vi "Write.vi"(8 "Error In":errorcluster, 9 "Data":u8[](array[numeric]), 10 "Command":u8, 11 "EZ430-Chronos Config":T1) -> (0 "Error Out":errorcluster, 3 "EZ430-Chronos Config":T1)   [LabVIEW 2011, in "LVH-EZ430.lvlib"]
uses:
  <vilib>/LabVIEW Hacker/LabVIEW Interface for EZ430-Chronos/LVH-EZ430.lvlib
  <vilib>/LabVIEW Hacker/LabVIEW Interface for EZ430-Chronos/Private/Type Defs/EZ430-Chronos Ref.ctl
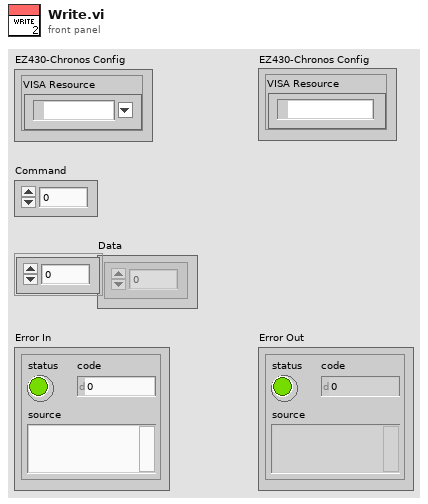
[diagram p1: front panel]
types:
  T1 = typedef "LVH-EZ430.lvlib/EZ430-Chronos Ref.ctl" = cluster{"VISA Resource":refnum<visa-resource-name>}
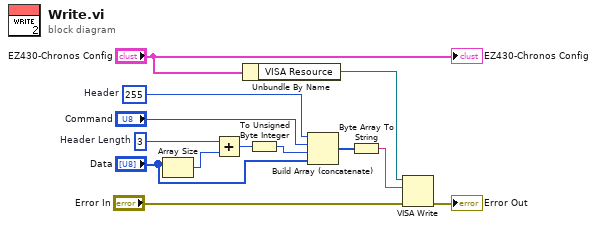
[diagram p0: block diagram]
diagram:
  w10 = 3  # Header Length
  w13 = u8 255  # Header
  n1 = Array Size(array="Data") -> (size(s)=w11:i32)
  n2 = Add(x=w10, y=w11) -> (x+y=w9:i32)
  n3 = Unbundle By Name("EZ430-Chronos Config") -> ("VISA Resource"=w5:refnum<visa-resource-name>)
  n4 = To Unsigned Byte Integer(number=w9) -> (unsigned 8bit integer=w8:u8)
  n5 = Build Array (concatenate)(w13, "Command", w8, "Data") -> (w6:u8[])
  n6 = Byte Array To String(unsigned byte array=w6) -> (string=w4:string)
  n7 = VISA Write(VISA resource name=w5, write buffer=w4, error in (no error)="Error In") -> (error out=→"Error Out":errorcluster)  [unwired: 2 out]
  "EZ430-Chronos Config" <- "EZ430-Chronos Config"
